vi "Read Assert Factory.vi"(8 "error in (no error)":errorcluster) -> (0 "error out":errorcluster, 3 "Test Assert Factory":refnum<class "Test Assert Factory.lvclass">)   [LabVIEW 2013, in "Caraya.lvlib" / "Assert Factory Manager.lvclass"]
doc: "Returns the currently registered Assert Factory implementaiton."
uses:
  Assert Factory Manager.lvclass
  Test Assert Factory/Test Assert Factory.lvclass
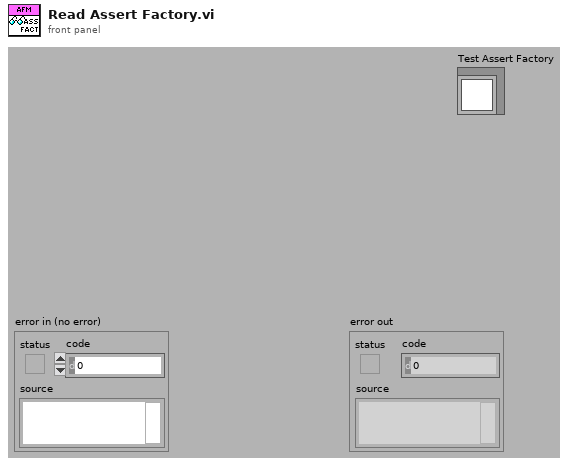
[diagram p1: front panel]
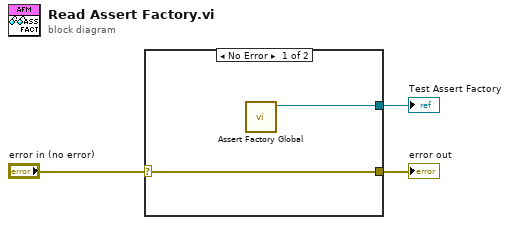
[diagram p0: block diagram]
diagram:
  n1 = case shown="No Error" "error in (no error)" {
    selector: "error in (no error)" -> [w4 w6]
    tunnel: [w5 _] -> w3
    tunnel: [w4 w6] -> w1
    frame No Error {
      n2 = call "Assert Factory Global.vi"() -> ("Test Assert Factory out"=w5:refnum<class "Test Assert Factory.lvclass">)  [unwired: 9 in, 2 out]
    }
    frame Error {
    }
  }
  "Test Assert Factory" <- w3
  "error out" <- w1
